vi "Is_File.vi"(8 "error in (no error)":errorcluster, 11 "IB_Tree_Item_Proj_File in":refnum<class "IB_Tree_Item_Proj_File.lvclass">) -> (0 "error out":errorcluster, 2 "file?":bool, 3 "IB_Tree_Item_Proj_File out":refnum<class "IB_Tree_Item_Proj_File.lvclass">)   [LabVIEW 2020, in "IB_Tree_Item_Proj_File.lvclass"]
uses:
  <vilib>/AppBuilder/IB_Classes/Tree_Item_Proj_File/IB_Tree_Item_Proj_File.lvclass
  <vilib>/AppBuilder/IB_Classes/Tree_Item_Proj_File/IB_Tree_Item_Proj_File.lvclass/IB_Tree_Item_Proj_File.ctl
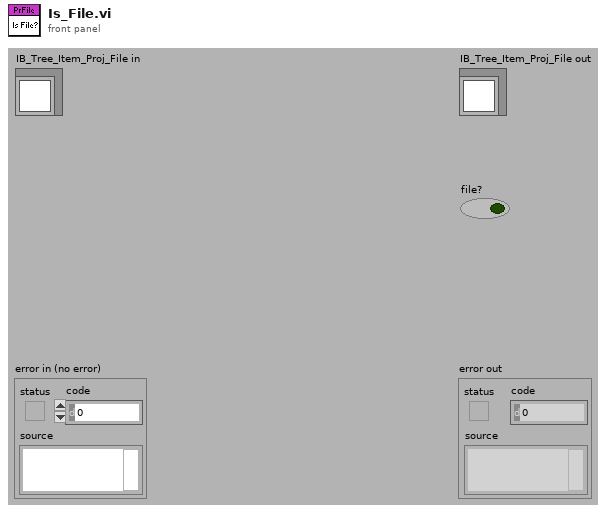
[diagram p1: front panel]
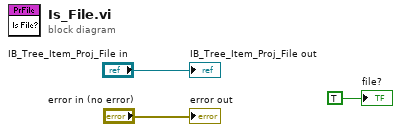
[diagram p0: block diagram]
diagram:
  "error out" <- "error in (no error)"
  "IB_Tree_Item_Proj_File out" <- "IB_Tree_Item_Proj_File in"
  "file?" <- TRUE ("file?")
